vi "Compress.vi"(8 "错误输入":errorcluster, 11 "String":string) -> (0 "错误输出":errorcluster, 1 "Ratio":dbl, 3 "Compressed String":string)   [LabVIEW 2012, in "GZip.lvlib"]
uses:
  GZip.lvlib
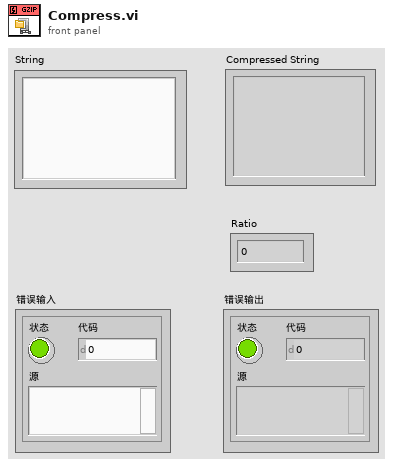
[diagram p1: front panel]
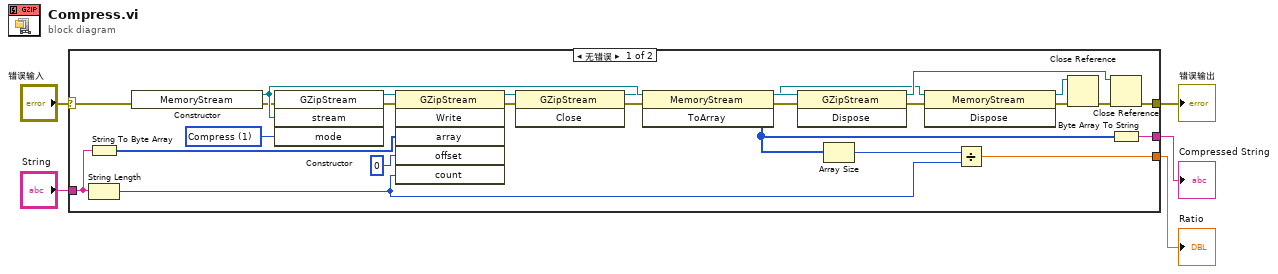
[diagram p0: block diagram]
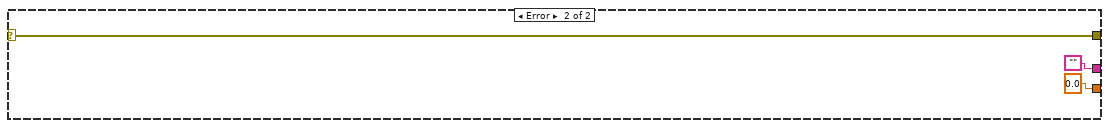
[diagram p2: hidden frame]
diagram:
  n1 = case shown="无错误" "错误输入" {
    selector: "错误输入" -> [w18 w34]
    tunnel: "String" -> [w28 _]
    tunnel: [w13 w34] -> w1
    tunnel: [w7 0.0] -> w2
    tunnel: [w6 "" ("string")] -> w3
    frame No Error {
      w21 = 1 items=["Decompress", "Compress"] ("mode")
      n2 = String To Byte Array(string=w28) -> (unsigned byte array=w19:u8[])
      n3 = String Length(string=w28) -> (length=w8:i32)
      n4 = constructor class="MemoryStream"(error in=w18) -> (reference out=w24:refnum<k24>, error out=w20:errorcluster)  [unwired: 2 in, 1 out]
      n5 = constructor class="GZipStream"(error in=w20, "stream"=w24, "mode"=w21) -> (reference out=w22:refnum<k24>, error out=w23:errorcluster)  [unwired: 2 in, 3 out]
      n6 = invoke class="GZipStream" method="Write"(reference=w22, error in=w23, "array"=w19, "offset"=0, "count"=w8) -> (reference out=w30:refnum<k24>, error out=w25:errorcluster)  [unwired: 1 in, 4 out]
      n7 = invoke class="GZipStream" method="Close"(reference=w30, error in=w25) -> (reference out=w12:refnum<k24>, error out=w26:errorcluster)  [unwired: 1 in, 1 out]
      n8 = invoke class="MemoryStream" method="ToArray"(reference=w24, error in=w26) -> (reference out=w11:refnum<k24>, error out=w31:errorcluster, "ToArray"=w10:u8[])  [unwired: 1 in]
      n9 = invoke class="GZipStream" method="Dispose"(reference=w12, error in=w31) -> (reference out=w14:refnum<k24>, error out=w29:errorcluster)  [unwired: 1 in, 1 out]
      n10 = Array Size(array=w10) -> (size(s)=w9:i32)
      n11 = invoke class="MemoryStream" method="Dispose"(reference=w11, error in=w29) -> (reference out=w16:refnum<k24>, error out=w17:errorcluster)  [unwired: 1 in, 1 out]
      n12 = Divide(x=w9, y=w8) -> (x/y=w7:dbl)
      n13 = Close Reference(reference=w16, error in (no error)=w17) -> (error out=w15:errorcluster)
      n14 = Close Reference(reference=w14, error in (no error)=w15) -> (error out=w13:errorcluster)
      n15 = Byte Array To String(unsigned byte array=w10) -> (string=w6:string)
    }
    frame Error {
    }
  }
  "错误输出" <- w1
  "Compressed String" <- w3
  "Ratio" <- w2
